vi "Add PV Value.vi"(5 "is read only? (F)":bool, 7 "PV name":string, 8 "error in":errorcluster, 10 "NT Base in":refnum<class "NT Base.lvclass">, 11 "Source in":refnum<class "Source.lvclass">) -> (0 "error out":errorcluster, 2 "NT Base out":refnum<class "NT Base.lvclass">, 3 "Source out":refnum<class "Source.lvclass">)   [LabVIEW 2020, in "PV Access.lvlib" / "PVA Server.lvlib" / "Source.lvclass"]
uses:
  Source.lvclass
  PV Data/NT Base/NT Base.lvclass
  PV Data/PV Data/PV Data.lvclass
  Source.lvclass/Source.ctl
  PV Access.lvlib
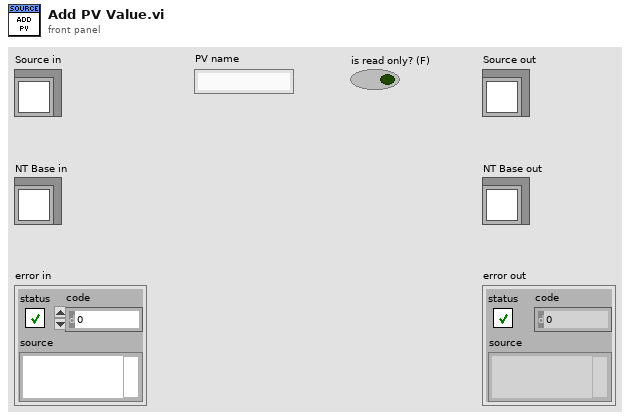
[diagram p1: front panel]
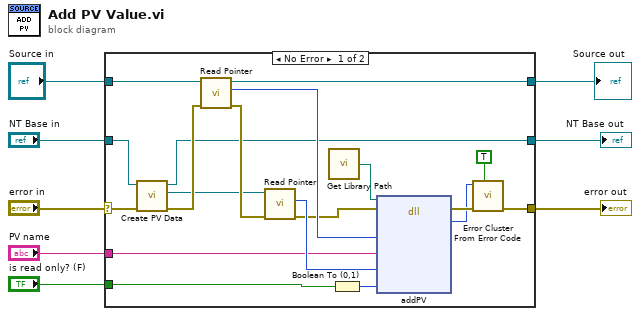
[diagram p0: block diagram]
diagram:
  n1 = case shown="No Error" "error in" {
    selector: "error in" -> [w15 w30]
    tunnel: [w19 w30] -> w7
    tunnel: [w17 w29] -> w5
    tunnel: "Source in" -> [w18 w29]
    tunnel: "PV name" -> [w25 _]
    tunnel: "NT Base in" -> [w14 w28]
    tunnel: [w12 w28] -> w2
    tunnel: "is read only? (F)" -> [w9 _]
    frame No Error {
      n2 = call-dynamic "Create PV Data.vi"("error in (no error)"=w15, "NT Base in"=w14) -> ("error out"=w13:errorcluster, "PV Data out"=w11:refnum<class "PV Data.lvclass">, "NT Base out"=w12:refnum<class "NT Base.lvclass">)  [unwired: 7 in]
      n3 = call-dynamic "Read Pointer.vi"("error in (no error)"=w13, "Pointer Base in"=w18) -> ("error out"=w27:errorcluster, "Pointer"=w24:i64, "Pointer Base out"=w17:refnum<class "Source.lvclass">)  [unwired: 7 in]
      n4 = call-dynamic "Read Pointer.vi"("error in (no error)"=w27, "Pointer Base in"=w11) -> ("error out"=w16:errorcluster, "Pointer"=w26:i64)  [unwired: 7 in, 1 out]
      n5 = call "Get Library Path.vi"() -> ("Path"=w23:path)  [unwired: 1 in]
      n6 = Boolean To (0,1)(Boolean=w9) -> (0, 1=w10:i16)
      n7 = dll-call lib="?" fn="addPV"(path in=w23, error in=w16, "source"=w24, "pv_name"=w25, "value"=w26, "read only?"=w10) -> (error out=w21:errorcluster, "ret_code"=w20:i32)  [unwired: 5 in, 1 out]
      n8 = call <vilib>:"Error Cluster From Error Code.vi"("show call chain? (False)"=TRUE, "error in (no error)"=w21, "error code (0)"=w20) -> ("error out"=w19:errorcluster)  [unwired: 6 in]
    }
    frame Error {
    }
  }
  "error out" <- w7
  "Source out" <- w5
  "NT Base out" <- w2
